vi "uA__daq_Set_Power_supply_for_DUT.vi"(8 "error in":errorcluster, 10 "DUT Voltage Selector":enum16{"3.8VDC", "2.9VDC", "3.7VDC", "4.0VDC"}(ring), 11 "USB DAQ":tag) -> (0 "error out":errorcluster)   [LabVIEW 2015]
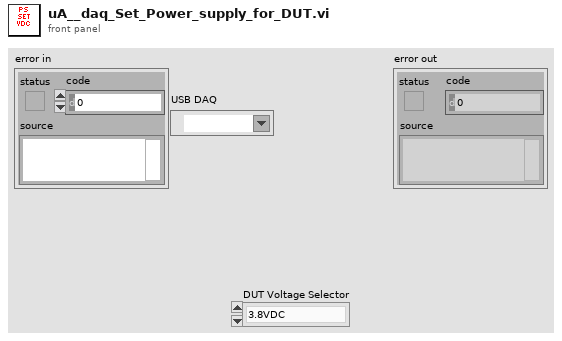
[diagram p1: front panel]
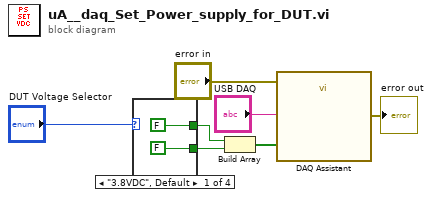
[diagram p0: block diagram]
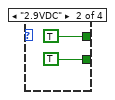
[diagram p2: hidden frame]
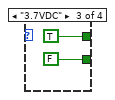
[diagram p3: hidden frame]
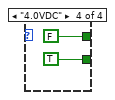
[diagram p4: hidden frame]
diagram:
  n1 = case shown="\"3.8VDC\", Default" "DUT Voltage Selector" {
    tunnel: [FALSE TRUE FALSE TRUE] -> w4
    tunnel: [FALSE TRUE TRUE FALSE] -> w5
    frame "3.8VDC", Default {
    }
    frame "2.9VDC" {
    }
    frame "3.7VDC" {
    }
    frame "4.0VDC" {
    }
  }
  n2 = Build Array(w5, w4) -> (w3:bool[])
  n3 = call "DAQ Assistant"("data"=w3, "error in"="error in", "device name"="USB DAQ") -> ("error out"=→"error out":errorcluster)  [unwired: 15 in, 1 out]
